vi "Actor Core.vi"(8 "error in":errorcluster, 11 "StopEnabledActor in":refnum<class "StopEnabledActor.lvclass">) -> (0 "error out":errorcluster, 3 "Actor out":refnum<class "Actor.lvclass">)   [LabVIEW 2017, in "StopEnabledActor.lvclass"]
doc: "(<B>Filename</B>: Actor Framework.lvlib:Actor.lvclass:Actor Core.vi)\n\nReceives messages to the actor, reacts to them, and initiates any error handling that may shut the actor down.\n\nDescendant classes may override this VI to append parallel tasks for the actor to complete while it handles messages. Overrides use the Call Parent Method node."
uses:
  StopEnabledActor.lvclass
  <vilib>/ActorFramework/Actor/Actor.lvclass
  StopEnabledActor.lvclass/StopEnabledActor.ctl
panel:
  out "Boolean":bool
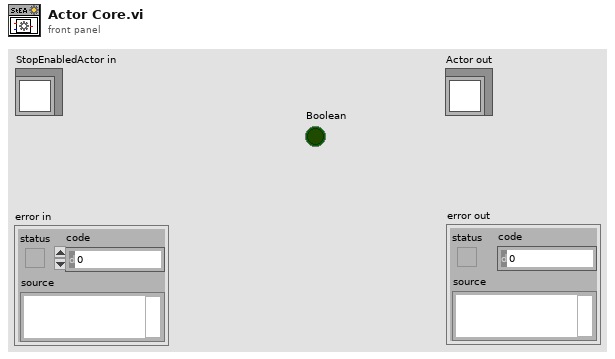
[diagram p1: front panel]
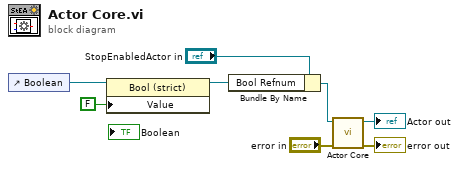
[diagram p0: block diagram]
diagram:
  n1 = control-ref of="Boolean"() -> (w3:refnum<vi>)
  n2 = property class="Bool (strict)"(reference=w3, "Value"=FALSE) -> (reference out=w2:refnum<vi>)  [unwired: 1 in, 1 out]
  n3 = Bundle By Name(cluster="StopEnabledActor in", "Bool Refnum"=w2) -> (w4:refnum<class "StopEnabledActor.lvclass">)
  n4 = call-parent "Actor Core.vi"("error in"="error in", "Actor in"=w4) -> ("error out"=→"error out":errorcluster, "Actor out"=→"Actor out":refnum<class "Actor.lvclass">)  [unwired: 8 in]
